vi "数据流写入.vi"() -> ()   [LabVIEW 2016, in "质控单元V4.lvlib"]
panel:
  out "读取方url":string
  in  "停止":bool
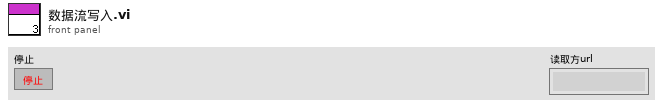
[diagram p1: front panel]
types:
  T1 = typedef "质控单元V4.lvlib/数据流类型.ctl" = cluster{"cmd":enum16{"start", "stop"}, "data":variant}
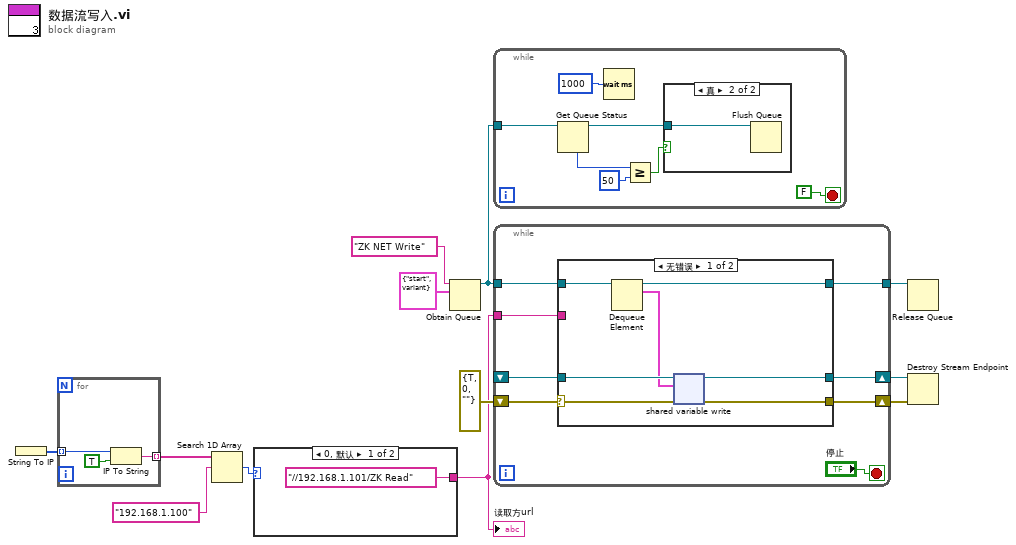
[diagram p0: block diagram]
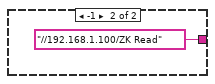
[diagram p2: hidden frame]
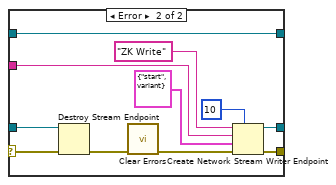
[diagram p4: hidden frame]
diagram:
  n1 = String To IP() -> (0:w6:u32[])  [unwired: 1 in]
  n2 = for {
    tunnel: w6 -> [w15] mode=indexing
    tunnel: [w13] -> w5 mode=indexing
    n3 = IP To String(1:TRUE ("句点符号？(F)"), 2:w15) -> (0:w13:string)
  }
  n4 = Search 1D Array(1D array=w5, element="192.168.1.100" ("元素")) -> (index of element=w3:i32)  [unwired: 1 in]
  n5 = case shown="0, 默认" w3 {
    tunnel: ["//192.168.1.101/ZK Read" ("读取方url") "//192.168.1.100/ZK Read" ("读取方url")] -> w2
    frame 0, Default {
    }
    frame -1 {
    }
  }
  "读取方url" <- w2
  n6 = Obtain Queue(name (unnamed)="ZK NET Write" ("名称（未命名）"), element data type=T1 {"cmd"=enum."start", "data"=variant} ("簇")) -> (queue out=w7:refnum<queue>)  [unwired: 3 in, 2 out]
  n7 = while {
    tunnel: w7 -> [w24]
    stop <- FALSE stop-if-true
    n8 = Get Queue Status(queue=w24) -> (queue out=w20:refnum<queue>, # elements in queue=w23:i32)  [unwired: 2 in, 6 out]
    n9 = Wait (ms)(milliseconds to wait=u32 1000 ("等待时间（毫秒）")) -> ()  [unwired: 1 out]
    n10 = Greater Or Equal?(x=w23, y=50) -> (x >= y?=w21:bool)
    n11 = case shown="真" w21 {
      tunnel: w20 -> [_ w25]
      frame False {
      }
      frame True {
        n12 = Flush Queue(queue=w25) -> ()  [unwired: 1 in, 3 out]
      }
    }
  }
  n13 = while {
    shift-right: [w33] -> w8
    shift-left: errorcluster {"status"=TRUE, "code"=0, "source"=""} ("error out") -> [w32]
    shift-right: [w31] -> w9
    shift-left: _ -> [w30]
    tunnel: w7 -> [w28]
    tunnel: [w27] -> w10
    tunnel: w2 -> [w26]
    stop <- "停止" stop-if-true
    n14 = case shown="无错误" w32 {
      selector: w32 -> [w39 w48]
      tunnel: [w37 w50] -> w33
      tunnel: [w38 w49] -> w31
      tunnel: w30 -> [w40 w47]
      tunnel: w28 -> [w36 w43]
      tunnel: [w34 w43] -> w27
      tunnel: w26 -> [_ w42]
      frame No Error {
        n15 = Dequeue Element(queue=w36) -> (queue out=w34:refnum<queue>, element=w35:T1)  [unwired: 2 in, 2 out]
        n16 = shared-variable-write(w40, w39, w35) -> (w38:refnum<k21>, w37:errorcluster)  [unwired: 1 in, 1 out]
      }
      frame Error {
        n17 = Destroy Stream Endpoint(8:w48, 11:w47) -> (0:w46:errorcluster)
        n18 = call <vilib>:"Clear Errors.vi"("error in (no error)"=w46) -> ("error out"=w45:errorcluster)  [unwired: 5 in, 1 out]
        n19 = Create Network Stream Writer Endpoint(7:10 ("写入方缓冲大小"), 8:w45, 9:T1 {"cmd"=enum."start", "data"=variant} ("簇"), 10:w42, 11:"ZK Write" ("写入方名称")) -> (0:w50:errorcluster, 3:w49:refnum<k21>)  [unwired: 2 in]
      }
    }
  }
  n20 = Release Queue(queue=w10) -> ()  [unwired: 2 in, 3 out]
  n21 = Destroy Stream Endpoint(8:w8, 11:w9) -> ()  [unwired: 1 out]
